vi "Test Bench.vi"() -> ()   [LabVIEW 2020]
uses:
  Door Controller/Doors Closed/Doors Closed.lvclass
  C:/Program Files/National Instruments/LabVIEW 2020/vi.lib/ActorFramework/Actor/Actor.lvclass
  <vilib>/ActorFramework/Message Enqueuer/Message Enqueuer.lvclass/Message Enqueuer.ctl
  <vilib>/ActorFramework/Message Enqueuer/Enqueue.vi
  Door Controller/Door Controller Messages/Close Door Msg/Close Door Msg.lvclass
  C:/Program Files/National Instruments/LabVIEW 2020/vi.lib/ActorFramework/Message/Message.lvclass
  Door Controller/Door Controller Messages/Open Door Msg/Open Door Msg.lvclass
  <vilib>/ActorFramework/Stop Msg/Stop Msg.lvclass
  <vilib>/ActorFramework/Message Priority Queue/Priority Enqueue.vi
  <vilib>/ActorFramework/Actor/Actor.lvclass
panel:
  in  "Emergency Declared":bool
  in  "Close Doors":bool
  in  "Open Doors":bool
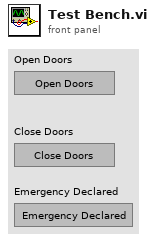
[diagram p1: front panel]
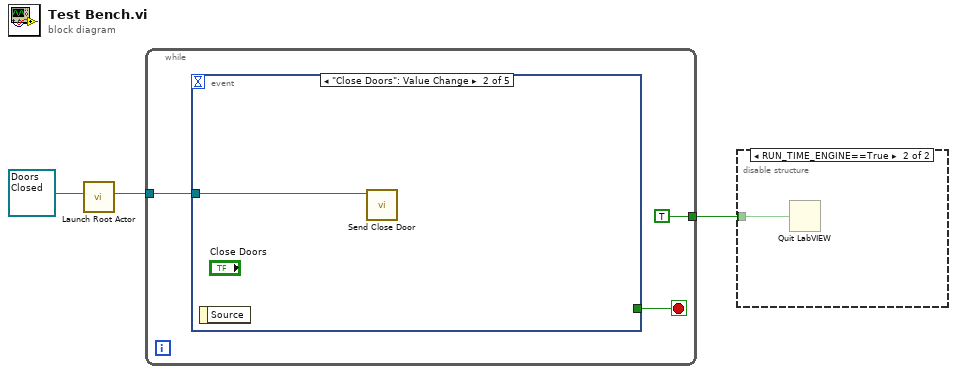
[diagram p0: block diagram]
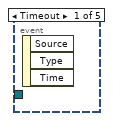
[diagram p3: hidden frame]
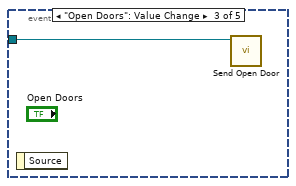
[diagram p4: hidden frame]
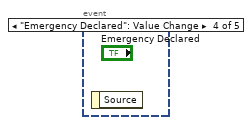
[diagram p5: hidden frame]
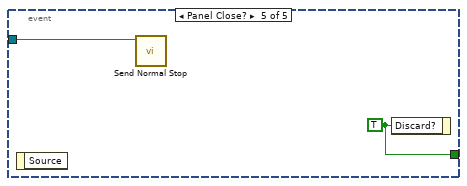
[diagram p6: hidden frame]
diagram:
  n1 = call <vilib>:"Launch Root Actor.vi"("Actor"=refnum<class "Doors Closed.lvclass"> refnum ("Door Controller.lvlib:Doors Closed.lvclass")) -> ("Actor's Enqueuer"=w2:refnum<class "Message Enqueuer.lvclass">)  [unwired: 9 in, 1 out]
  n2 = while {
    tunnel: w2 -> [w5]
    tunnel: [TRUE] -> w1
    stop <- w6 stop-if-true
    n3 = event shown="[1] \"Close Doors\": Value Change" {
      selector: _ -> [_ _ _ _ _]
      dyn-events: _ -> [_ _ _ _ _]
      timeout: _ -> [_ _ _ _ _]
      tunnel: [_ _ _ _ w10] -> w6
      tunnel: w5 -> [_ w7 w8 _ w9]
      event Timeout {
        n4 = event-data() -> ()  [unwired: 1 in, 3 out]
      }
      event "Close Doors": Value Change {
        n5 = event-data() -> ()  [unwired: 1 in, 1 out]
        n6 = call "Send Close Door.vi"("Message Enqueuer"=w7) -> ()  [unwired: 9 in, 2 out]
      }
      event "Open Doors": Value Change {
        n7 = event-data() -> ()  [unwired: 1 in, 1 out]
        n8 = call "Send Open Door.vi"("Message Enqueuer"=w8) -> ()  [unwired: 9 in, 2 out]
      }
      event "Emergency Declared": Value Change {
        n9 = event-data() -> ()  [unwired: 1 in, 1 out]
      }
      event Panel Close? {
        w10 = TRUE ("Discard?")
        n10 = event-data() -> ()  [unwired: 1 in, 1 out]
        n11 = call <vilib>:"Send Normal Stop.vi"("Message Enqueuer"=w9) -> ()  [unwired: 10 in, 1 out]
        n12 = event-data("Discard?"=w10) -> ()  [unwired: 1 in, 1 out]
      }
    }
  }
  n13 = disable-structure shown="RUN_TIME_ENGINE==True" {
    disable-tunnel: w1 -> [_ w11]
    frame condition #0 (active) {
    }
    frame condition #1 {
      n14 = Quit LabVIEW(quit? (T)=w11) -> ()
    }
  }
